vi "Lab1.vi"() -> ()   [LabVIEW 2016]
uses:
  <vilib>/addons/Control Design/_Model Construction/Data Typedefs.llb/CD Variables.ctl
  <vilib>/addons/Control Design/_Model Construction/Data Typedefs.llb/CD Time Info.ctl
  <vilib>/addons/Control Design/_Model Construction/Model Creation.llb/Model Creation SubVI/cd_Create Symbolic Transfer Function Model.vi
  <vilib>/addons/Control Design/_Model Interconnection/Model Interconnection.llb/Model Interconnection SubVI/cd_Series (TF and TF).vi
  <vilib>/addons/Control Design/_Model Construction/Model Creation.llb/Model Creation SubVI/cd_Create Transfer Function Model.vi
  <vilib>/addons/Control Design/_Model Interconnection/Model Interconnection.llb/Model Interconnection SubVI/cd_Feedback (TF and TF).vi
  <vilib>/addons/Control Design/_Time Response Analysis/Time Response.llb/Time Response subVI/cd_Step Response (Transfer Function).vi
  <vilib>/addons/Control Design/_Model Construction/NI_LinSys_Model Creation.lvlib
  <vilib>/addons/Control Design/_Model Interconnection/NI_CD_Model Interconnection.lvlib
  <vilib>/addons/Control Design/_Time Response Analysis/NI_CD_Time Response.lvlib
  <vilib>/addons/Control Design/_Model Construction/NI_LinSys_Data Typedefs.lvlib
panel:
  in  "stop":bool
  out "Step Response Graph":cluster{"time":dbl[], dbl[]}[](graph)
  in  "Time Range":T1={"t0"=-1.0, "dt"=-1.0, "tf"=-1.0} {"dt" format="%#.6g"; "tf" format="%#.6g"; "t0" format="%#.6g"}
  in  "Variables 2":T2 {"Value" format="%.2f"}
  in  "Variables":T2 {"Value" format="%_5e"}
  in  "Symbolic Denominator 2":string[](array[string])
  in  "Symbolic Denominator":string[](array[string])
  in  "Symbolic Numerator 2":string[](array[string])
  in  "Symbolic Numerator":string[](array[string])
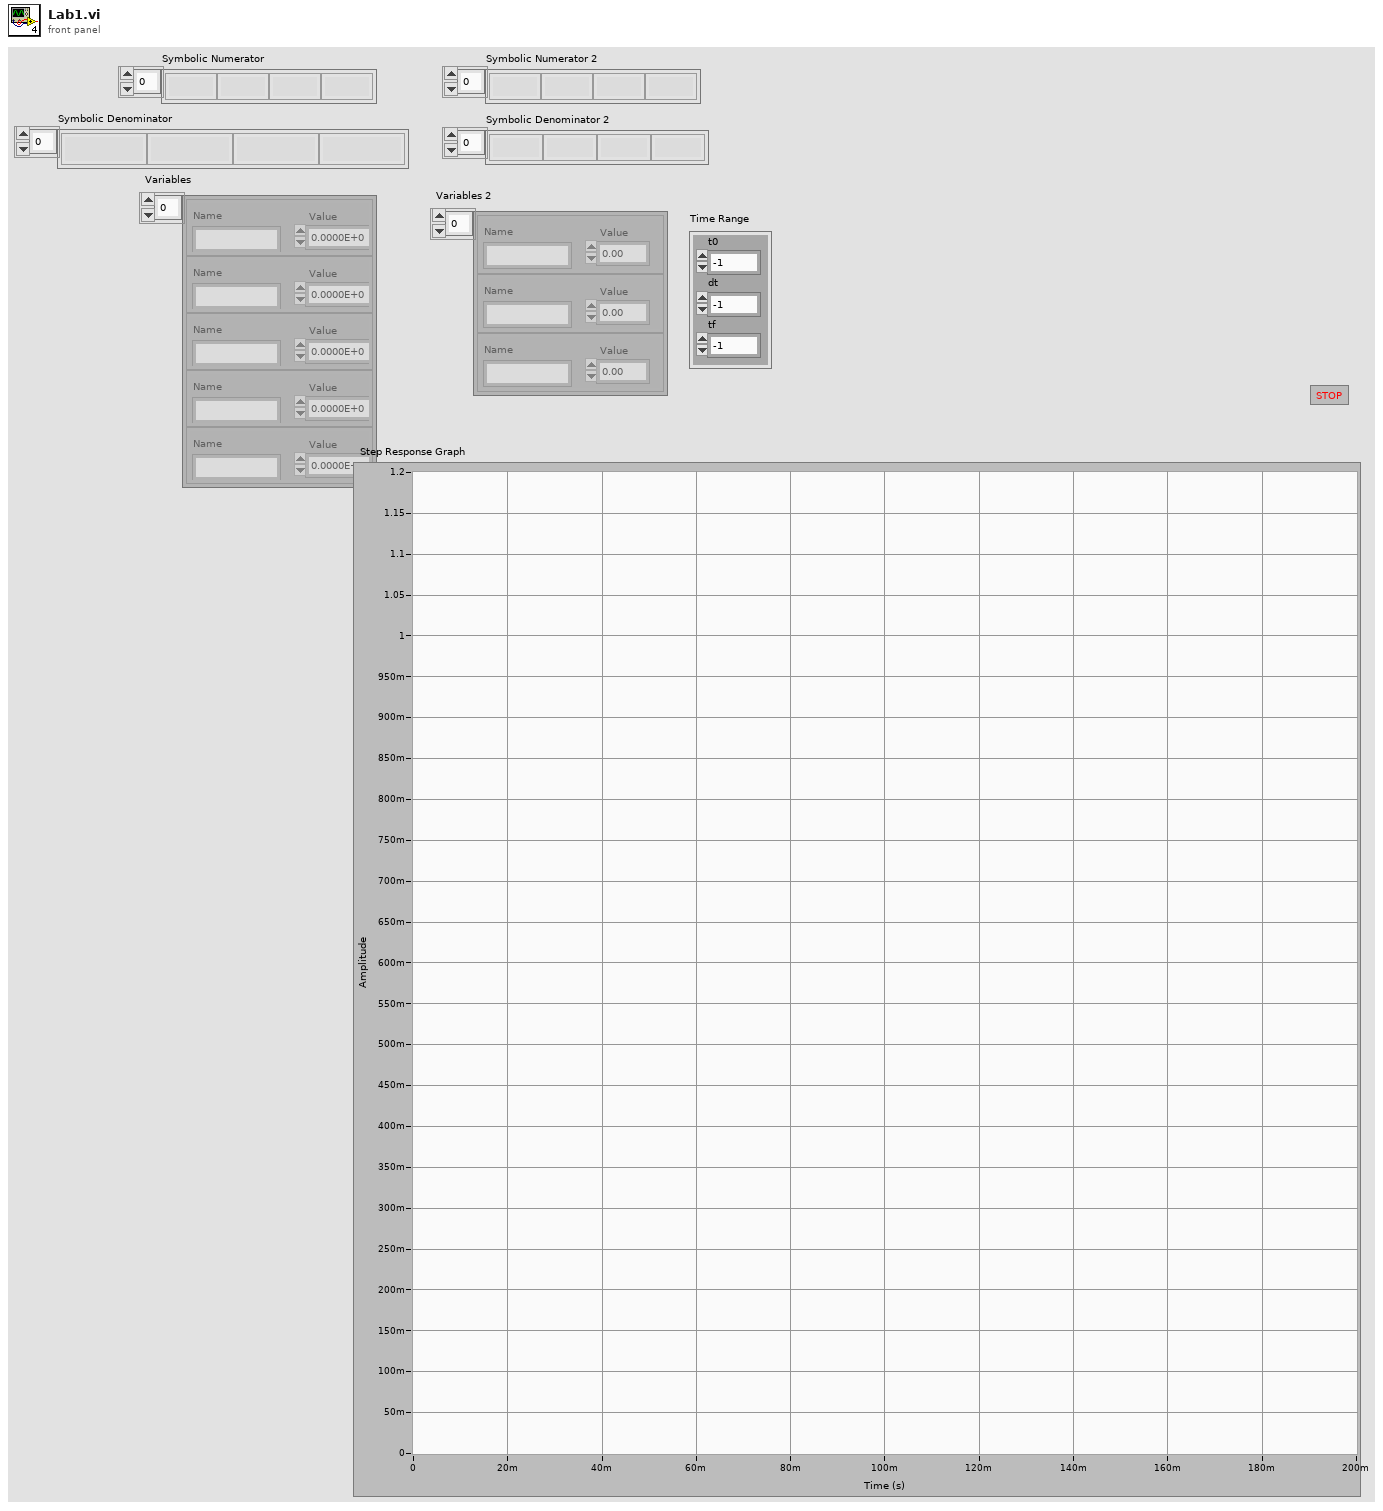
[diagram p1: front panel]
types:
  T1 = typedef "NI_LinSys_Data Typedefs.lvlib/CD Time Info.ctl" = cluster{"t0":dbl, "dt":dbl, "tf":dbl}
  T2 = typedef "NI_LinSys_Data Typedefs.lvlib/CD Variables.ctl" = cluster{"Name":string, " Value":dbl}[]
  T3 = typedef "NI_LinSys_Model Typedefs.lvlib/CD Transfer Function Model (MIMO).ctl" = cluster{"properties":T4, "transfer function(s)":T5[][]}
  T4 = typedef "NI_LinSys_Model Typedefs.lvlib/CD General Elements.ctl" = cluster{"Model name":string, "Input names":string[], "Output names":string[], "Input Delays":dbl[], "Output Delays":dbl[], "Sampling Time":dbl, "Notes":string}
  T5 = typedef "NI_LinSys_Model Typedefs.lvlib/CD Transfer Function Model (SISO).ctl" = cluster{"Numerator":dbl[], "Denominator":dbl[], "delay":dbl}
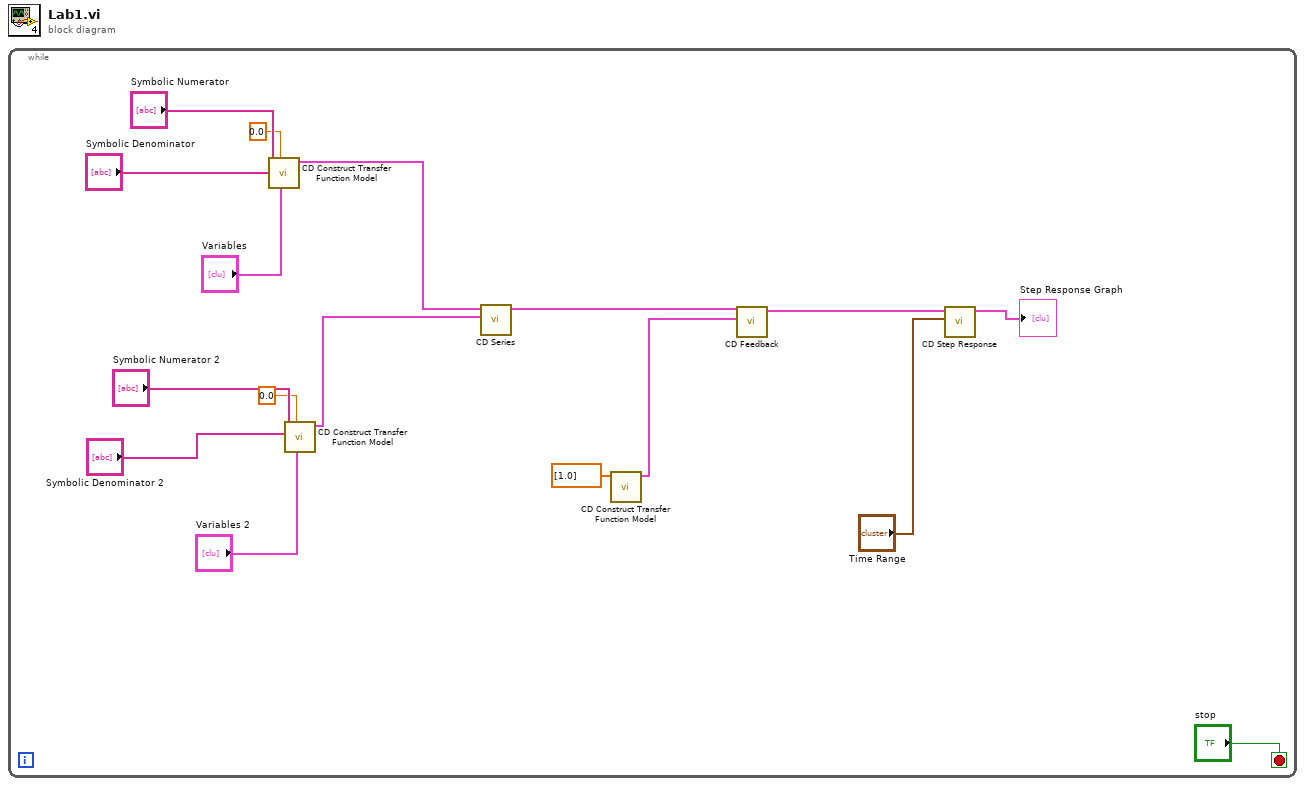
[diagram p0: block diagram]
diagram:
  n1 = while {
    stop <- "stop" stop-if-true
    n2 = call-poly <vilib>:"CD Construct Transfer Function Model.vi"("Variables"="Variables", "Sampling Time (s)"=0.0, "Symbolic Denominator"="Symbolic Denominator", "Symbolic Numerator"="Symbolic Numerator") -> ("Transfer Function Model"=w8:T3)  [unwired: 6 in, 1 out]
    n3 = call-poly <vilib>:"CD Construct Transfer Function Model.vi"("Variables"="Variables 2", "Sampling Time (s)"=0.0, "Symbolic Denominator"="Symbolic Denominator 2", "Symbolic Numerator"="Symbolic Numerator 2") -> ("Transfer Function Model"=w9:T3)  [unwired: 6 in, 1 out]
    n4 = call-poly <vilib>:"CD Series.vi"("Model 2"=w9, "Model 1"=w8) -> ("Series Model"=w7:T3)  [unwired: 8 in, 1 out]
    n5 = call-poly <vilib>:"CD Construct Transfer Function Model.vi"("Numerator"=dbl[] [1.0]) -> ("Transfer Function Model"=w5:T3)  [unwired: 9 in, 1 out]
    n6 = call-poly <vilib>:"CD Feedback.vi"("Model 2"=w5, "Model 1"=w7) -> ("Closed-Loop Model"=w2:T3)  [unwired: 8 in, 1 out]
    n7 = call-poly <vilib>:"CD Step Response.vi"("Time Range"="Time Range", "Transfer Function Model"=w2) -> ("Step Response Graph"=→"Step Response Graph":cluster{"time":dbl[], dbl[]}[])  [unwired: 7 in, 2 out]
  }
